vi "Set VI Reentrancy.vi"(8 "error in (no error)":errorcluster, 10 "Reentrancy Type":T1(ring), 11 "vi ref in":refnum<vi>) -> (0 "error out":errorcluster, 3 "vi ref out":refnum<vi>)   [LabVIEW 2017, in "Build Automation.lvlib"]
uses:
  Build Automation.lvlib
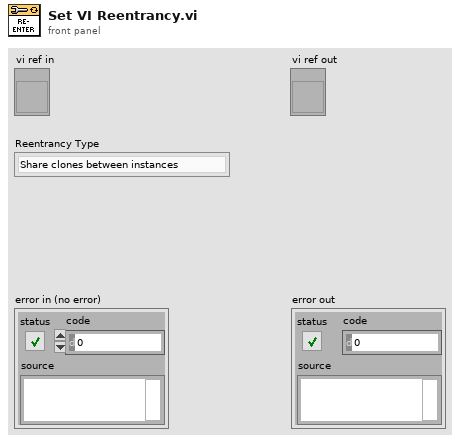
[diagram p1: front panel]
types:
  T1 = enum16{"Share clones between instances", "Preallocate clone for each instance"}
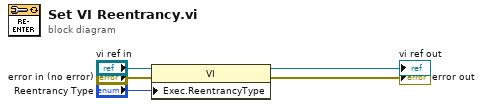
[diagram p0: block diagram]
diagram:
  n1 = property class="VI"(reference="vi ref in", error in="error in (no error)", "Exec.ReentrancyType"="Reentrancy Type") -> (reference out=→"vi ref out":refnum<vi>, error out=→"error out":errorcluster)
